vi "Waveform_Analog2Digital.vi"(8 "error in (no error)":errorcluster, 10 "\"Binary waveform\"":waveform(dbl)(graph)) -> (0 "error out":errorcluster, 3 "Digital signal":digitalwaveform(graph))   [LabVIEW 2025]
doc: "This Vi convert an analog waveform into a digital waveform"
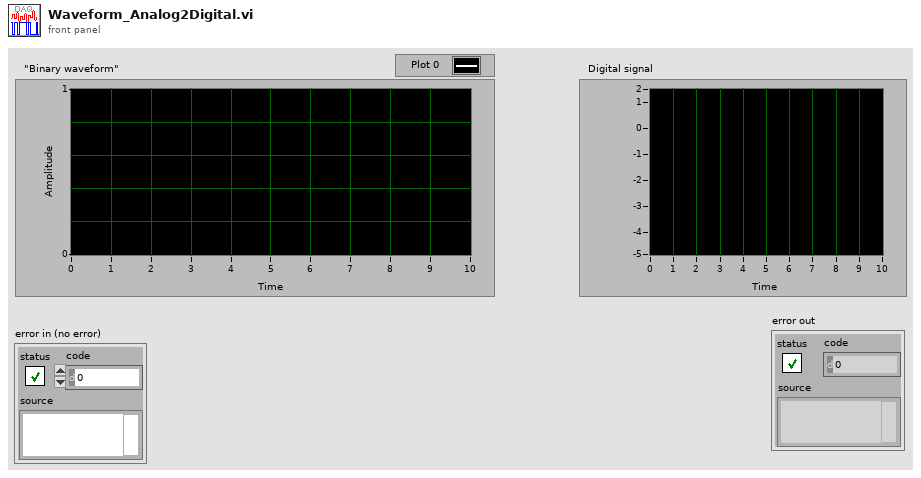
[diagram p1: front panel]
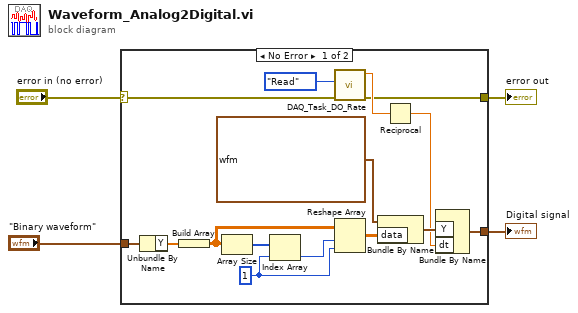
[diagram p0: block diagram]
diagram:
  n1 = case shown="No Error" "error in (no error)" {
    selector: "error in (no error)" -> [w7 w20]
    tunnel: [w19 _] -> w4
    tunnel: "\"Binary waveform\"" -> [w18 _]
    tunnel: [w6 w20] -> w1
    frame No Error {
      w14 = 1 ("index")
      n2 = Unbundle By Name(w18) -> ("Y"=w10:dbl[])
      n3 = Build Array(w10) -> (w11:dbl[][])
      n4 = Array Size(array=w11) -> (size(s)=w12:i32[])
      n5 = Index Array(array=w12, index=w14) -> (element=w13:i32)
      n6 = call "DAQ_Task_DO_Rate.vi"("error in"=w7, "Action"=enum16{"Write", "Read"}."Read") -> ("error out"=w6:errorcluster, "DO_Rate"=w8:dbl)  [unwired: 8 in]
      n7 = Reshape Array(w11, w13, w14) -> (w15:dbl[][])
      n8 = Bundle By Name(cluster=digitaldata {"transitions"=[], "data"=[]} ("Type of waveform I need to create"), "data"=w15) -> (w17:digitaldata)
      n9 = Reciprocal(x=w8) -> (1/x=w5:dbl)
      n10 = Bundle By Name("Y"=w17, "dt"=w5) -> (w19:digitalwaveform)  [unwired: 1 in]
    }
    frame Error {
    }
  }
  "Digital signal" <- w4
  "error out" <- w1
